vi "2_test_2摄像头读取设别.vi"() -> ()   [LabVIEW 2020]
uses:
  <vilib>/vision/driver/NI_Vision_Acquisition_Software.lvlib
panel:
  in  "停止":bool
  out "Image":T1(plugin-control)
  in  "IMAQdx Session":refnum<k21>
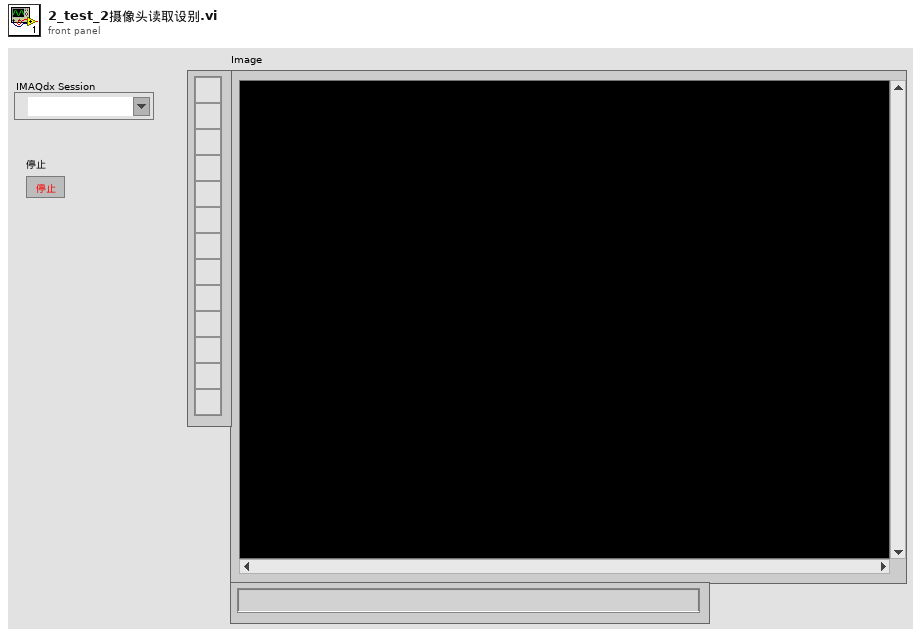
[diagram p1: front panel]
types:
  T1 = typedef "IMAQ Image.ctl" = refnum<image>
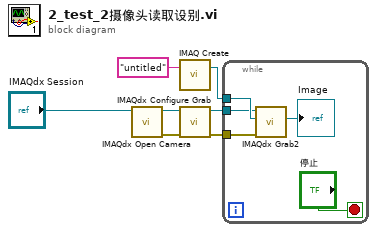
[diagram p0: block diagram]
diagram:
  n1 = call <vilib>:"IMAQdx Open Camera.vi"("Session In"="IMAQdx Session") -> ("error out"=w6:errorcluster, "Session Out"=w7:refnum<k21>)  [unwired: 9 in]
  n2 = call "IMAQ Create"("Image Name"="untitled") -> ("New Image"=w2:T1)  [unwired: 4 in, 1 out]
  n3 = call <vilib>:"IMAQdx Configure Grab.vi"("error in"=w6, "Session In"=w7) -> ("error out"=w3:errorcluster, "Session Out"=w1:refnum<k21>)  [unwired: 8 in]
  n4 = while {
    tunnel: w3 -> [w12]
    tunnel: w2 -> [w11]
    tunnel: w1 -> [w10]
    stop <- "停止" stop-if-true
    n5 = call <vilib>:"IMAQdx Grab2.vi"("error in"=w12, "Image In"=w11, "Session In"=w10) -> ("Image Out"=→"Image":T1)  [unwired: 5 in, 3 out]
  }
